vi "SetCurveParams.vi"(6 "VarPar list":string[](array[string]), 7 "AllowDef":bool, 8 "error in (no error)":errorcluster caption="entrée d'erreur (pas d'erreur)", 9 "VarParams":string[][](array[string]), 10 "CurveSetupsIn":T1[](array[typedef]), 11 "CurveNames":string[](array[string])) -> (0 "error out":errorcluster caption="sortie d'erreur", 2 "CurveSetupsOut":T1[](array[typedef]))   [LabVIEW 2019, in "Interface.lvclass"]
uses:
  Interface.lvclass
  CurveSetup.ctl
  <userlib>/GenProg/ArrayTo1DString.vi
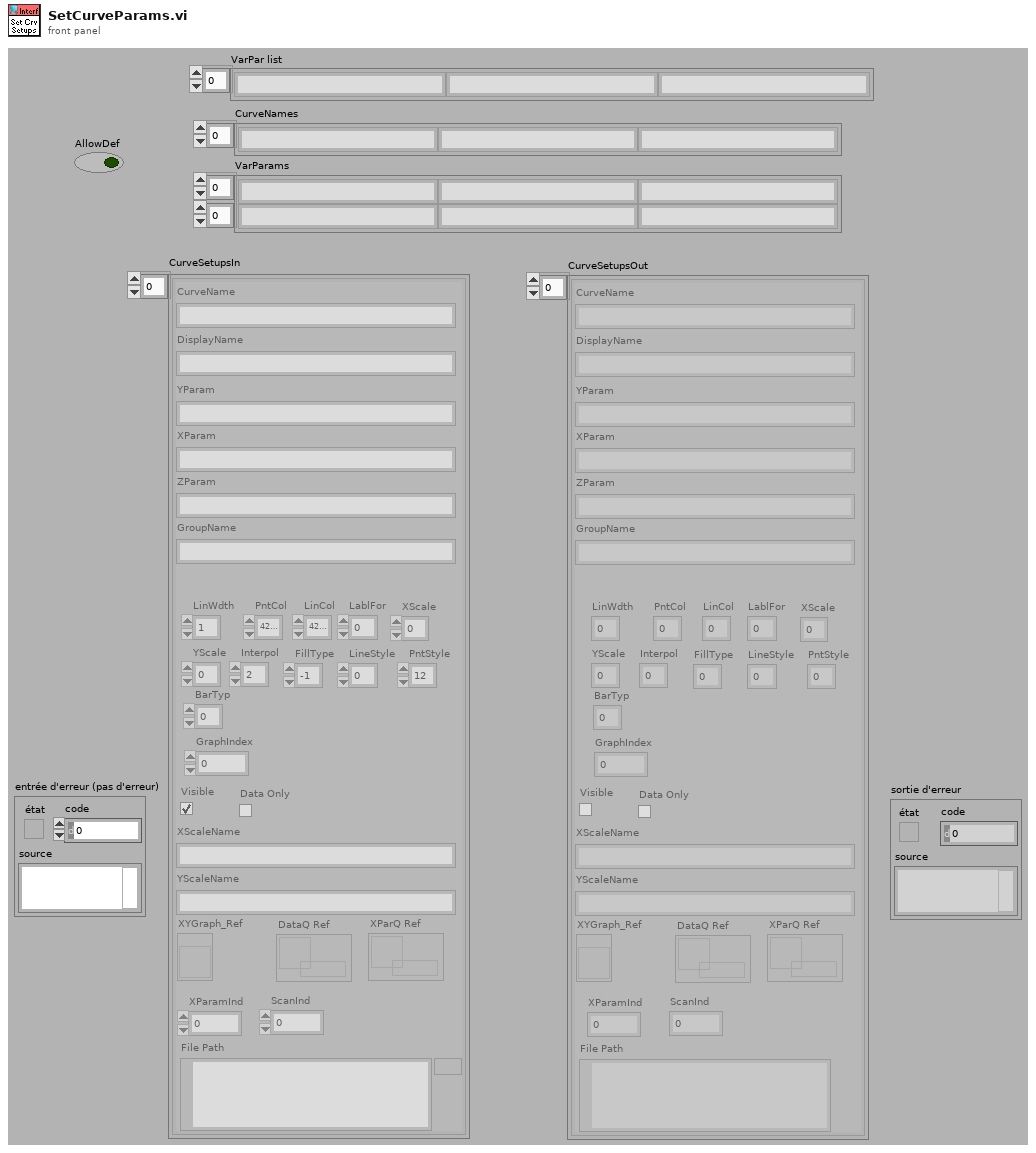
[diagram p1: front panel]
types:
  T1 = typedef "Interface.lvclass/CurveSetup.ctl" = cluster{"CurveName":string, "YParam":string, "XParam":string, "ZParam ":string, "GroupName":string, "LinWdth":u8, "PntCol":u32, "LinCol":u32, "LablFor":u8, "XScale":u32, "YScale":u32, "Interpol":u8, "DisplayName":string, "FillType":i16, "LineStyle":u8, "PntStyle":u8, "BarTyp":u8, "GraphIndex":i32, "Visible":bool, "XScaleName":string, "YScaleName":string, "XYGraph_Ref":refnum<vi>, "Data Only":bool, "DataQ Ref":refnum<queue>, "XParQ Ref":refnum<queue>, "XParamInd":i32, "ScanInd":i32, "File Path":path}
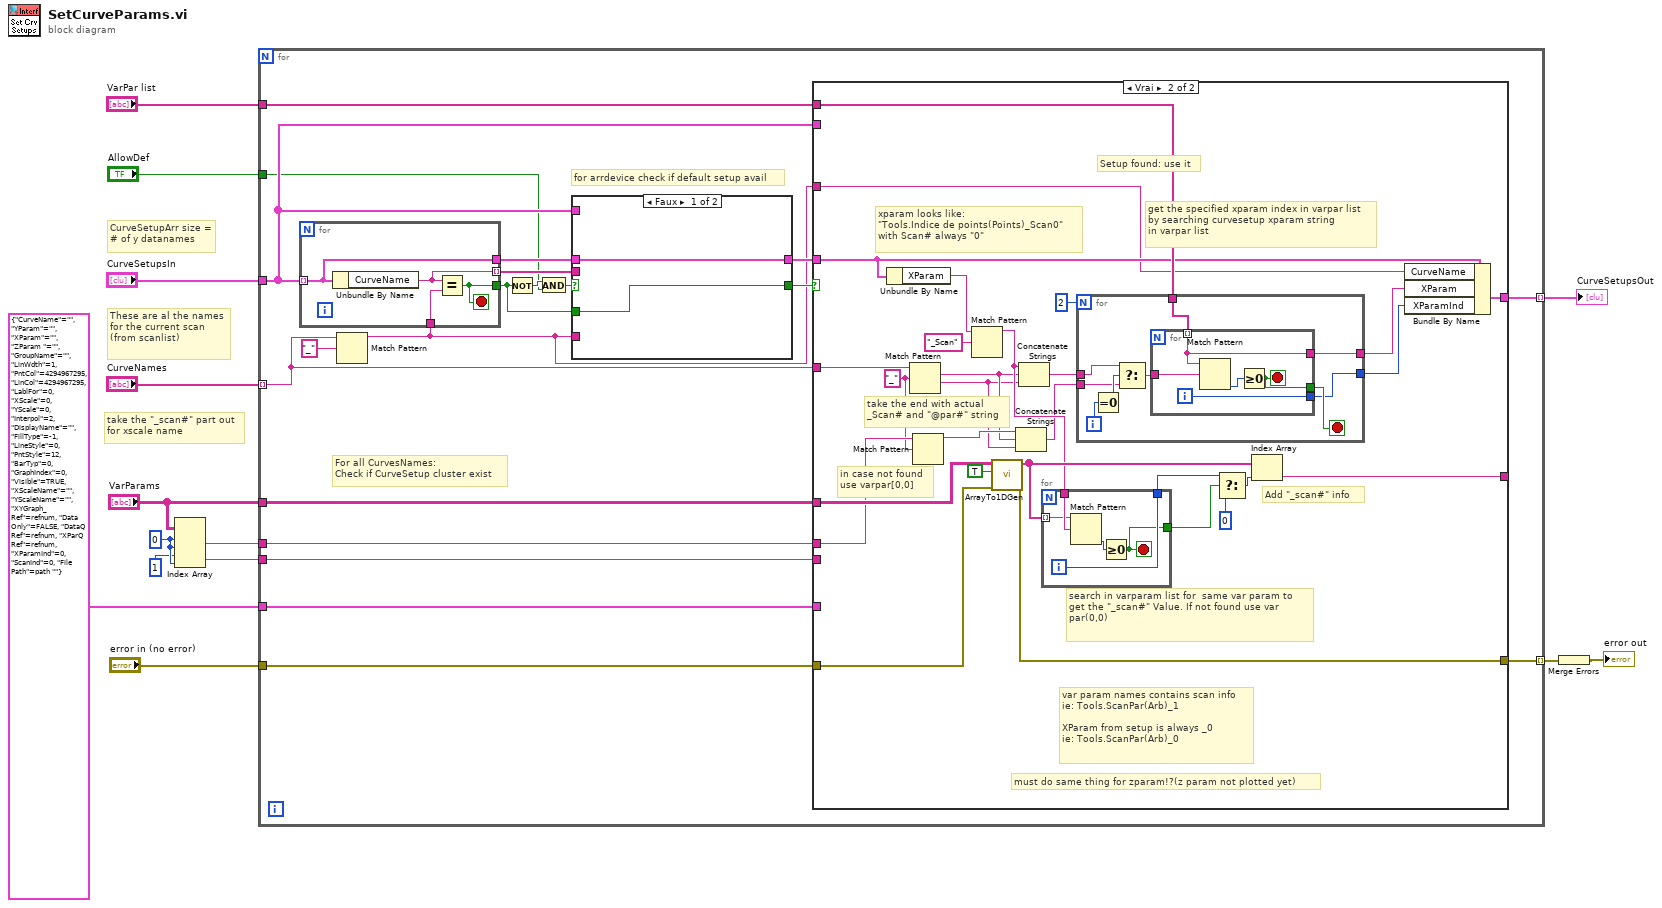
[diagram p0: block diagram]
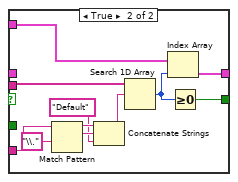
[diagram p2: hidden frame]
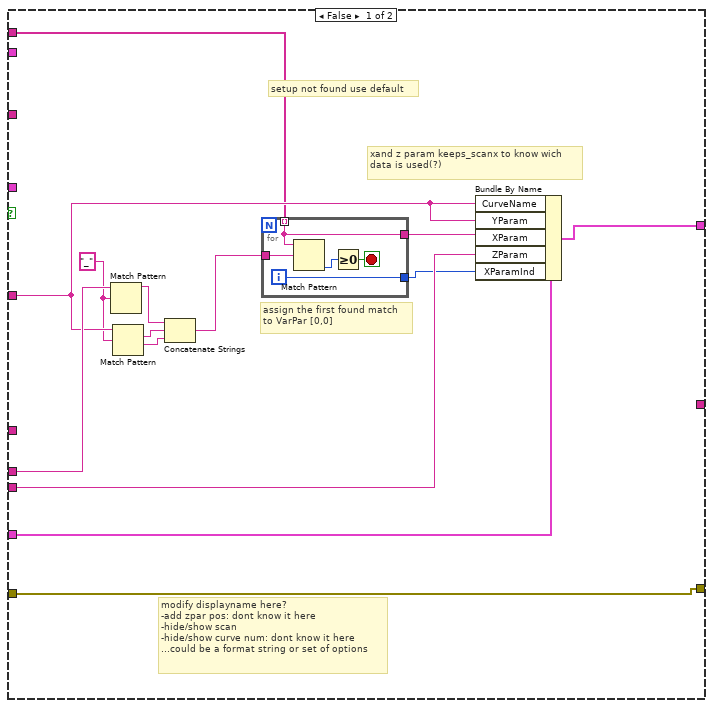
[diagram p3: hidden frame]
diagram:
  w9 = 0 ("indice (ligne)")
  # "take the \"_scan#\" part out\nfor xscale name"
  # "These are al the names for the current scan (from scanlist)"
  # "CurveSetupArr size = # of y datanames"
  n1 = Index Array(array="VarParams", index (row) #1=w9, index (col) #1=w9, index (row) #2=1 ("indice (ligne)"), index (col) #2=w9) -> (element #1=w5:string, element #2=w6:string)
  n2 = for {
    tunnel: "CurveNames" -> [w29] mode=indexing
    tunnel: "CurveSetupsIn" -> [w20]
    tunnel: [w34] -> w11 mode=indexing
    tunnel: T1 {"CurveName"="", "YParam"="", "XParam"="", "ZParam "="", "GroupName"="", "LinWdth"=1, "PntCol"=4294967295, "LinCol"=4294967295, "LablFor"=0, "XScale"=0, "YScale"=0, "Interpol"=2, "DisplayName"="", "FillType"=-1, "LineStyle"=0, "PntStyle"=12, "BarTyp"=0, "GraphIndex"=0, "Visible"=TRUE, "XScaleName"="", "YScaleName"="", "XYGraph_Ref"=refnum, "Data Only"=FALSE, "DataQ Ref"=refnum, "XParQ Ref"=refnum, "XParamInd"=0, "ScanInd"=0, "File Path"=path ""} ("CurveParam") -> [w33]
    tunnel: "VarParams" -> [w32]
    tunnel: "error in (no error)" -> [w31]
    tunnel: w5 -> [w28]
    tunnel: w6 -> [w27]
    tunnel: [w26] -> w4 mode=indexing
    tunnel: "VarPar list" -> [w25]
    tunnel: "AllowDef" -> [w17]
    # "for arrdevice check if default setup avail"
    # "For all CurvesNames:\nCheck if CurveSetup cluster exist"
    n3 = Match Pattern(string=w29, regular expression="_" ("expression régulière")) -> (before substring=w15:string)  [unwired: 1 in, 3 out]
    n4 = for {
      tunnel: w20 -> [w116] mode=indexing
      tunnel: [w117] -> w16
      tunnel: [w116] -> w23
      tunnel: w15 -> [w115]
      tunnel: [w114] -> w21 mode=indexing
      stop <- w117 stop-if-true
      n5 = Unbundle By Name(w116) -> ("CurveName"=w114:string)
      n6 = Equal?(x=w114, y=w115) -> (x = y?=w117:bool)
    }
    n7 = Not(x=w16) -> (.not. x?=w19:bool)
    n8 = And(x=w19, y=w17) -> (x .and. y?=w18:bool)
    n9 = case shown="Faux" w18 {
      tunnel: [w36 w37] -> w24
      tunnel: w23 -> [w36 _]
      tunnel: [w35 w41] -> w22
      tunnel: w15 -> [_ w43]
      tunnel: w21 -> [_ w40]
      tunnel: w20 -> [_ w38]
      tunnel: w16 -> [w35 _]
      frame False {
      }
      frame True {
        n10 = Match Pattern(string=w43, regular expression="\\.") -> (before substring=w46:string, match substring=w45:string)  [unwired: 1 in, 2 out]
        n11 = Concatenate Strings(w46, w45, "Default" ("string")) -> (w42:string)
        n12 = Search 1D Array(1D array=w40, element=w42) -> (index of element=w39:i32)  [unwired: 1 in]
        n13 = Index Array(array=w38, index=w39) -> (element=w37:T1)
        n14 = Greater Or Equal To 0?(x=w39) -> (x >= 0?=w41:bool)
      }
    }
    n15 = case shown="Vrai" w22 {
      tunnel: w24 -> [_ w76]
      tunnel: [w60 w94] -> w34
      tunnel: w33 -> [w61 _]
      tunnel: w32 -> [_ w93]
      tunnel: w31 -> [w58 w89]
      tunnel: w29 -> [w55 w77]
      tunnel: w28 -> [w56 w74]
      tunnel: w27 -> [w59 _]
      tunnel: [w58 w85] -> w26
      tunnel: w25 -> [w53 w84]
      tunnel: [_ w79] -> _
      tunnel: w20 -> [_ _]
      tunnel: w15 -> [_ w75]
      frame False {
        w48 = "_" ("regular expression")
        # "assign the first found match\nto VarPar [0,0]"
        # "xand z param keeps_scanx to know wich data is used(?)"
        # "modify displayname here?\n-add zpar pos: dont know it here\n-hide/show scan\n-hide/show curve num: dont know it here\n...could be a format string or set of options"
        # "setup not found use default"
        n16 = Match Pattern(string=w56, regular expression=w48) -> (before substring=w57:string)  [unwired: 1 in, 3 out]
        n17 = Match Pattern(string=w55, regular expression=w48) -> (match substring=w50:string, after substring=w49:string)  [unwired: 1 in, 2 out]
        n18 = Concatenate Strings(w57, w50, w49) -> (w52:string)
        n19 = for {
          tunnel: w53 -> [w64] mode=indexing
          tunnel: w52 -> [w66]
          tunnel: [w65] -> w54
          tunnel: [w64] -> w51
          i -> [w65]
          stop <- w62 stop-if-true
          n20 = Match Pattern(string=w64, regular expression=w66) -> (offset past match=w63:i32)  [unwired: 1 in, 3 out]
          n21 = Greater Or Equal To 0?(x=w63) -> (x >= 0?=w62:bool)
        }
        n22 = Bundle By Name(cluster=w61, "CurveName"=w55, "YParam"=w55, "XParam"=w51, "ZParam"=w59, "XParamInd"=w54) -> (w60:T1)
      }
      frame True {
        w73 = "_" ("regular expression")
        # "in case not found\nuse varpar[0,0]"
        # "get the specified xparam index in varpar list\nby searching curvesetup xparam string\nin varpar list"
        # "take the end with actual\n_Scan# and \"@par#\" string"
        # "var param names contains scan info\nie: Tools.ScanPar(Arb)_1\n\nXParam from setup is always _0\nie: Tools.ScanPar(Arb)_0"
        # "search in varparam list for  same var param to get the \"_scan#\" Value. If not found use var par(0,0)"
        # "must do same thing for zparam!?(z param not plotted yet)"
        # "xparam looks like:\n\"Tools.Indice de points(Points)_Scan0\"\nwith Scan# always \"0\""
        # "Add \"_scan#\" info"
        # "Setup found: use it"
        n23 = Unbundle By Name(w76) -> ("XParam"=w78:string)
        n24 = Match Pattern(string=w77, regular expression=w73) -> (match substring=w71:string, after substring=w70:string)  [unwired: 1 in, 2 out]
        n25 = Match Pattern(string=w74, regular expression=w73) -> (before substring=w72:string)  [unwired: 1 in, 3 out]
        n26 = Match Pattern(string=w78, regular expression="_Scan") -> (before substring=w81:string)  [unwired: 1 in, 3 out]
        n27 = call-poly <userlib>:"ArrayTo1DGen.vi"("ErrorIn(No Error)"=w89, "DelArrEnd(F)"=TRUE ("DelArrEnd"), "tableau"=w93) -> ("sortie d'erreur"=w85:errorcluster, "Array Out"=w90:string[])  [unwired: 6 in, 1 out]
        n28 = Concatenate Strings(w72, w71, w70) -> (w67:string)
        n29 = Concatenate Strings(w81, w71, w70) -> (w83:string)
        n30 = for {
          tunnel: w90 -> [w112] mode=indexing
          tunnel: w81 -> [w113]
          tunnel: [w110] -> w82
          tunnel: [w109] -> w88
          i -> [w110]
          stop <- w109 stop-if-true
          n31 = Match Pattern(string=w112, regular expression=w113) -> (offset past match=w111:i32)  [unwired: 1 in, 3 out]
          n32 = Greater Or Equal To 0?(x=w111) -> (x >= 0?=w109:bool)
        }
        n33 = for {
          N: 2 -> [_]
          tunnel: w84 -> [w103]
          tunnel: w83 -> [w98]
          tunnel: [w102] -> w80
          tunnel: [w96] -> w69
          tunnel: w67 -> [w95]
          i -> [w100]
          stop <- w101 stop-if-true
          n34 = Equal To 0?(x=w100) -> (x = 0?=w99:bool)
          n35 = Select(t=w98, s=w99, f=w95) -> (s? t:f=w97:string)
          n36 = for {
            tunnel: w103 -> [w106] mode=indexing
            tunnel: w97 -> [w108]
            tunnel: [w107] -> w96
            tunnel: [w106] -> w102
            tunnel: [w104] -> w101
            i -> [w107]
            stop <- w104 stop-if-true
            n37 = Match Pattern(string=w106, regular expression=w108) -> (offset past match=w105:i32)  [unwired: 1 in, 3 out]
            n38 = Greater Or Equal To 0?(x=w105) -> (x >= 0?=w104:bool)
          }
        }
        n39 = Select(t=w82, s=w88, f=0 ("cas faux")) -> (s? t:f=w87:i32)
        n40 = Index Array(array=w90, index=w87) -> (element=w79:string)
        n41 = Bundle By Name(cluster=w76, "CurveName"=w75, "XParam"=w80, "XParamInd"=w69) -> (w94:T1)
      }
    }
  }
  "CurveSetupsOut" <- w11
  n42 = Merge Errors(w4) -> (→"error out":errorcluster)
